vi "Init.vi"(8 "error in (no error)":errorcluster, 10 "Channel":i16, 11 "TrialBasedExperiment in":refnum<class "NatImExperiment.lvclass">) -> (0 "error out":errorcluster, 3 "TrialBasedExperiment out":refnum<class "NatImExperiment.lvclass">)   [LabVIEW 2012, in "NatImExperiment.lvclass"]
uses:
  NatImExperiment.lvclass
  Trial Based Experiment Statechart/PassiveExperiment/PassiveExperiment.lvclass
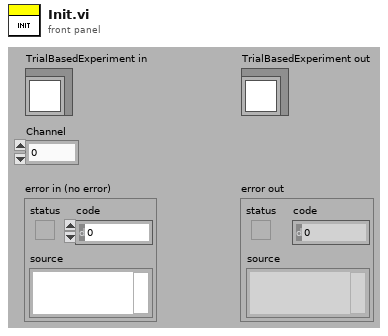
[diagram p1: front panel]
types:
  T1 = cluster{"Intertrial":dbl, "AcquireFixation":dbl, "HoldFixation":dbl, "DelayPeriod":dbl, "ResponsePeriod":dbl}
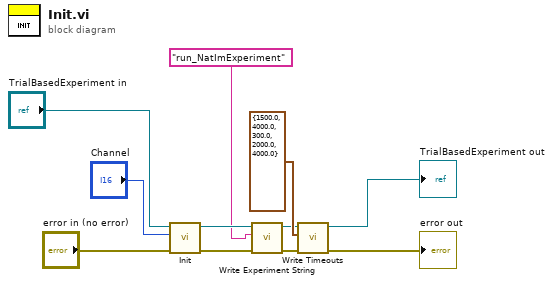
[diagram p0: block diagram]
diagram:
  n1 = call-parent "Init.vi"("error in (no error)"="error in (no error)", "Channel"="Channel", "TrialBasedExperiment in"="TrialBasedExperiment in") -> ("error out"=w2:errorcluster, "TrialBasedExperiment out"=w5:refnum<class "NatImExperiment.lvclass">)  [unwired: 7 in]
  n2 = call-dynamic "Write Experiment String.vi"("error in (no error)"=w2, "Experiment String"="run_NatImExperiment" ("string"), "TrialBasedExperiment in"=w5) -> ("error out"=w7:errorcluster, "TrialBasedExperiment out"=w6:refnum<class "NatImExperiment.lvclass">)  [unwired: 7 in]
  n3 = call-dynamic "Write Timeouts.vi"("error in (no error)"=w7, "Timeouts"=T1 {"Intertrial"=1500.0, "AcquireFixation"=4000.0, "HoldFixation"=300.0, "DelayPeriod"=2000.0, "ResponsePeriod"=4000.0}, "TrialBasedExperiment in"=w6) -> ("error out"=→"error out":errorcluster, "TrialBasedExperiment out"=→"TrialBasedExperiment out":refnum<class "NatImExperiment.lvclass">)  [unwired: 7 in]
